vi "step2 SolveUpperLeftCornerPiece.vi"(8 "error in (no error)":errorcluster, 11 "cube in":T1) -> (0 "error out":errorcluster, 3 "cube out":T1)   [LabVIEW 2011]
doc: "Rotate cube as necessary so that the top middle piece matches the desired start colour.\n\nNo transformations are done in this VI, the operations are loaded on the the operation queue bus."
uses:
  Typedef/cube.ctl
  Typedef/face.ctl
  Typedef/operation.ctl
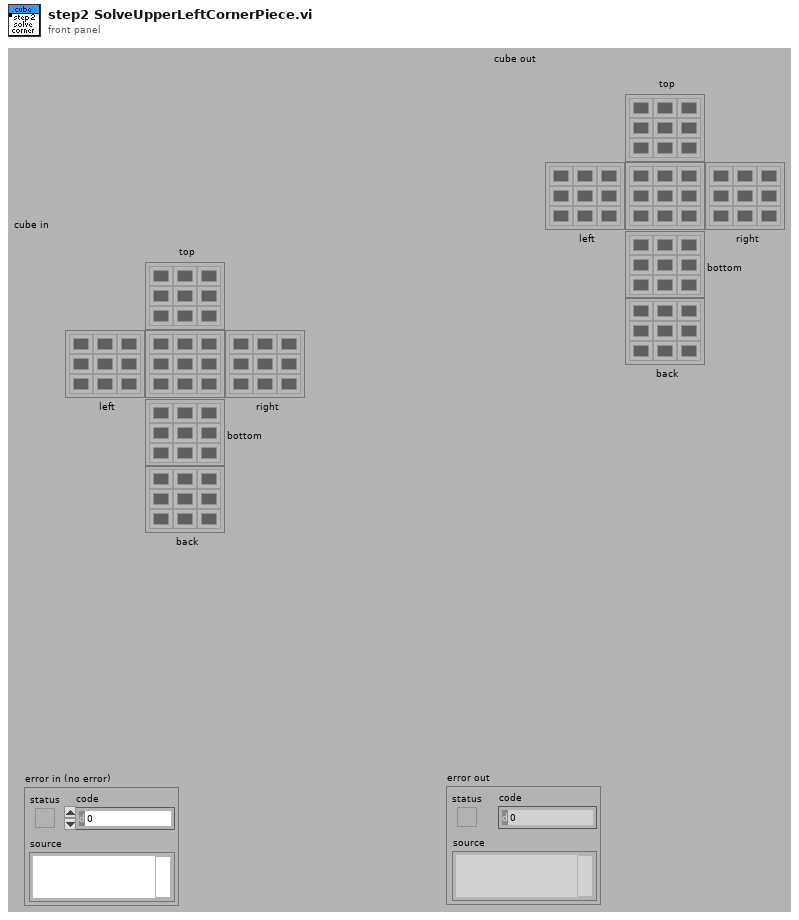
[diagram p1: front panel]
types:
  T1 = typedef "cube.ctl" = cluster{"top":T2, "left":T2, "right":T2, "bottom":T2, "back":T2, "front":T2}
  T2 = typedef "face.ctl" = u32[][]
  T3 = typedef "operation.ctl" = enum16{"nop", "T+", "T-", "F+", "F-", "L+", "L-", "R+", "R-", "B+", "B-", "<--", "-->", "^", "V"}
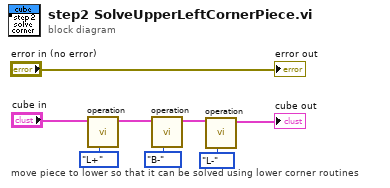
[diagram p0: block diagram]
diagram:
  # "move piece to lower so that it can be solved using lower corner routines"
  n1 = call "operation.vi"("operation"=operation."L+", "cube in"="cube in") -> ("cube out"=w4:T1)  [unwired: 8 in, 1 out]
  n2 = call "operation.vi"("operation"=operation."B-", "cube in"=w4) -> ("cube out"=w3:T1)  [unwired: 8 in, 1 out]
  n3 = call "operation.vi"("operation"=operation."L-", "cube in"=w3) -> ("cube out"=→"cube out":T1)  [unwired: 8 in, 1 out]
  "error out" <- "error in (no error)"
